vi "Distance Sensor-Dual.vi"() -> ()   [LabVIEW 2009]
uses:
  <vilib>/NXT/Block Support/NXT_InputPort.ctl
  <vilib>/NXT/Subs/LVHSConnector.ctl
  <vilib>/NXT/Dual Mode Library/Display/drawNumber.vi
  <vilib>/NXT/Dual Mode Library/Display/drawText.vi
  mindsensors.com LVEE Toolkit/Dual/Distance Sensor-DM.vi
panel:
  out "NXT dup":T1={"error"={"status"=FALSE, "code"=0, "source"=""}, "address"="", "NXT #"=-1, "Show Error"=TRUE}
  in  "NXT":T1={"error"={"status"=FALSE, "code"=0, "source"=""}, "address"="", "NXT #"=-1, "Show Error"=TRUE}
  in  "stop":bool
  out "Distance (mm)":ext(slide) scale=0.0..1600.0
  in  "Input Port":T2 items=["Port 1", "Port 2", "Port 3", "Port 4"]
  out "Distance":i16
  # "mm"
  # "mindsensors.com\nCopyright (c) 2009 by mindsensors.com\nEmail: info (<at>) mindsensors (<dot>) com\n\nThis program is free software. You can redistribute it and/or modify\nit under the terms of the GNU General Public License as published by the Free Software Foundation; version 3 of the License.\nRead the license at: http://www.gnu.org/licenses/gpl.txt"
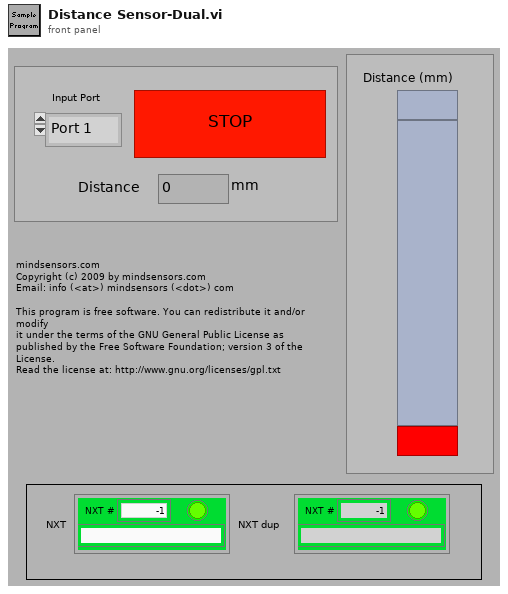
[diagram p1: front panel]
types:
  T1 = typedef "LVHSConnector.ctl" = cluster{"error":errorcluster, "address":string, "NXT #":i32, "Show Error":bool}
  T2 = typedef "NXT_InputPort.ctl" = u8
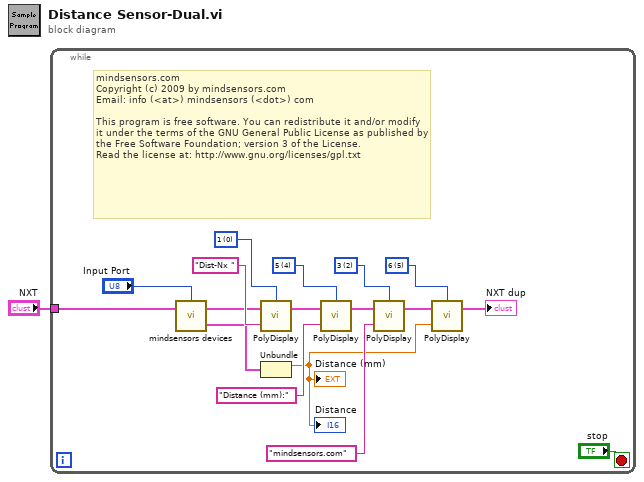
[diagram p0: block diagram]
diagram:
  n1 = while {
    tunnel: "NXT" -> [w17]
    stop <- "stop" stop-if-true
    w2 = i16 0 items=["1", "2", "3", "4", "5", "6", "7", "8"] ("Line")
    w9 = i16 5 items=["1", "2", "3", "4", "5", "6", "7", "8"] ("Line")
    w12 = i16 4 items=["1", "2", "3", "4", "5", "6", "7", "8"] ("Line")
    w14 = i16 2 items=["1", "2", "3", "4", "5", "6", "7", "8"] ("Line")
    # "mindsensors.com\nCopyright (c) 2009 by mindsensors.com\nEmail: info (<at>) mindsensors (<dot>) com\n\nThis program is free software. You can redistribute it and/or modify\nit under the terms of the GNU General Public License as published by\nthe Free Software Foundation; version 3 of the License.\nRead the license at: http://www.gnu.org/licenses/gpl.txt"
    n2 = call-poly "mindsensors devices.vi"("NXT"=w17, "Input Port"="Input Port") -> ("Output of Distance Sensor"=w10:cluster{"Distance Value":ext, "Status":bool}, "NXT dup"=w7:T1)  [unwired: 1 in]
    n3 = call-poly <vilib>:"PolyDisplay.vi"("Text"="Dist-Nx ", "NXT"=w7, "Line"=w2) -> ("NXT"=w6:T1)  [unwired: 1 in]
    n4 = Unbundle(w10) -> ("Distance Value"=w8:ext)  [unwired: 1 out]
    "Distance" <- w8
    "Distance (mm)" <- w8
    n5 = call-poly <vilib>:"PolyDisplay.vi"("Text"="Distance (mm):", "NXT"=w6, "Line"=w12) -> ("NXT"=w5:T1)  [unwired: 1 in]
    n6 = call-poly <vilib>:"PolyDisplay.vi"("Text"="mindsensors.com", "NXT"=w5, "Line"=w14) -> ("NXT"=w4:T1)  [unwired: 1 in]
    n7 = call-poly <vilib>:"PolyDisplay.vi"("number"=w8, "NXT"=w4, "Line"=w9) -> ("NXT"=→"NXT dup":T1)  [unwired: 1 in]
  }
